vi "Log Tester.vi"() -> ()   [LabVIEW 2015]
uses:
  Controls/QMH Fundamentals - Message Cluster.ctl
  Controls/Config_Stop Notifier Enum.ctl
  Controls/Control_Message Handling Cluster.ctl
  Controls/Control_M4X Connection.ctl
  Controls/Control_PXI-7854R FPGA Reference.ctl
  Controls/Control_Config Cluster.ctl
  Controls/Control_Config Unitherm Port.ctl
  Controls/Control_Config Simulate Values.ctl
  Controls/Control_Log Queue.ctl
  Controls/Control_Log Cluster.ctl
  Controls/Control_Log Time.ctl
  Controls/Control_Log Waveform Cluster.ctl
  Controls/Control_Log Analysis Cluster.ctl
  Controls/Control_Log Flag.ctl
  <vilib>/Waveform/WDTFileIO.llb/ Write Waveform to File.vi
  <vilib>/Waveform/WDTFileIO.llb/Export Waveforms To Spreadsheet File (1D).vi
panel:
  out "Saving Data":bool
  out "Time":timestamp
  in  "Simulate":bool
  out "Logging?":bool
  out "error out":errorcluster
  out "Measurements out":T1
  out "Waveform out":waveform(dbl)
  in  "error in (no error)":errorcluster
  in  "Log?":bool
  in  "Measurements in":T1
  in  "Waveform in":waveform(dbl)
  in  "stop":bool
  # "Real Values"
  # "Simulate"
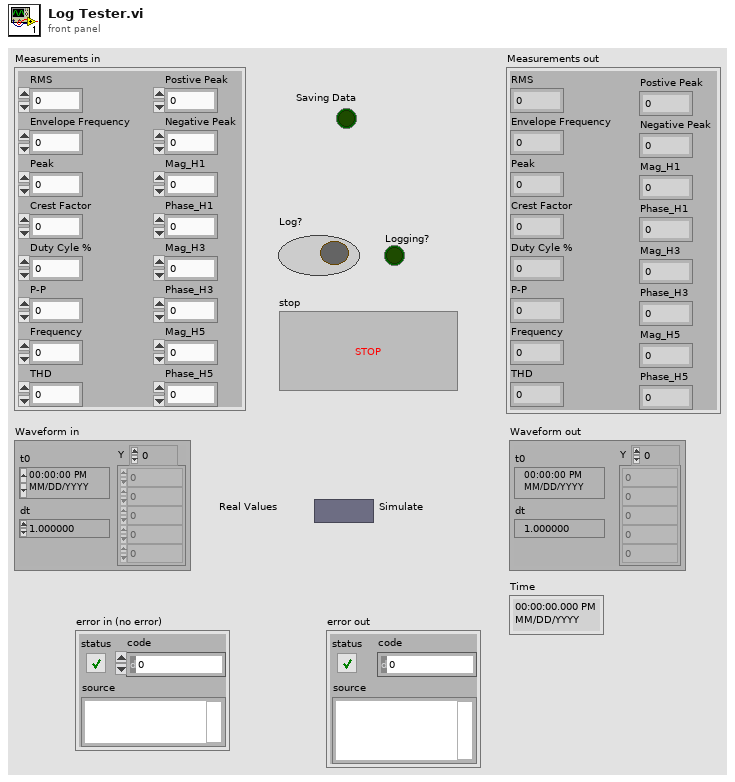
[diagram p1: front panel]
types:
  T1 = cluster{"RMS":dbl, "Envelope Frequency":dbl, "Peak":dbl, "Crest Factor":dbl, "Duty Cyle %":dbl, "P-P":dbl, "Frequency":dbl, "THD":dbl, "Postive Peak":dbl, "Negative Peak":dbl, "Mag_H1":dbl, "Phase_H1":dbl, "Mag_H3":dbl, "Phase_H3":dbl, "Mag_H5":dbl, "Phase_H5":dbl}
  T2 = enum16{"open", "open or create", "create or replace", "create", "open (read-only)"}
  T3 = cluster{"Time":timestamp, "Waveform":waveform(dbl), "Measurements":cluster{"RMS":dbl, "Envelope Frequency":dbl, "Peak":dbl, "Crest Factor":dbl, "Duty Cyle %":dbl, "P-P":dbl, "Frequency":dbl, "THD":dbl, "Postive Peak":dbl, "Negative Peak":dbl, "Mag_H1":dbl, "Phase_H1":dbl, "Mag_H3":dbl, "Phase_H3":dbl, "Mag_H5":dbl, "Phase_H5":dbl}}
  T4 = typedef "Config_Stop Notifier Enum.ctl" = enum16{"Initialize", "Read Notifier", "Notify", "Close"}
  T5 = cluster{"Log":bool, "Card Handle in":u32, "Simulate?":bool, "Measurements":cluster{"RMS":dbl, "Envelope Frequency":dbl, "Peak":dbl, "Crest Factor":dbl, "Duty Cyle %":dbl, "P-P":dbl, "Frequency":dbl, "THD":dbl, "Postive Peak":dbl, "Negative Peak":dbl, "Mag_H1":dbl, "Phase_H1":dbl, "Mag_H3":dbl, "Phase_H3":dbl, "Mag_H5":dbl, "Phase_H5":dbl}, "Waveform":waveform(dbl)}
  T6 = typedef "QMH Fundamentals - Message Cluster.ctl" = cluster{"Message":string, "Message Data":variant}
  T7 = typedef "Control_Message Handling Cluster.ctl" = cluster{"Fornax Connected?":refnum<vi>, "Unitherm Connected?":refnum<vi>, "M4X Connected?":refnum<vi>, "Unitherm Connect/Disconnect":refnum<vi>, "Fornax Connection":refnum<k5>, "UNITHERM Connection":refnum<visa-resource-name>, "M4X Connection":T8, "PXI-7854R FPGA Reference":T9, "PXI-7854R Connected?":refnum<vi>, "Fornax Connect/Disconnect":refnum<vi>, "7854 Connect/Disconnect":refnum<vi>, "M4X Connect/Disconnect":refnum<vi>, "Config Cluster":T10, "Log Queue":T13, "Log Analysis Cluster":T14, "Log Waveform Cluster":T15, "Log Time":T16, "Log Flag":T17}
  T8 = typedef "Control_M4X Connection.ctl" = u32
  T9 = typedef "Control_PXI-7854R FPGA Reference.ctl" = refnum<k20>
  T10 = typedef "Control_Config Cluster.ctl" = cluster{"Unitherm Port":T11, "Simulate Values":T12}
  T11 = typedef "Control_Config Unitherm Port.ctl" = string
  T12 = typedef "Control_Config Simulate Values.ctl" = bool
  T13 = typedef "Control_Log Queue.ctl" = refnum<queue>
  T14 = typedef "Control_Log Analysis Cluster.ctl" = cluster{"RMS":dbl, "Envelope Frequency":dbl, "Peak":dbl, "Crest Factor":dbl, "Duty Cyle %":dbl, "P-P":dbl, "Frequency":dbl, "THD":dbl, "Postive Peak":dbl, "Negative Peak":dbl, "Mag_H1":dbl, "Phase_H1":dbl, "Mag_H3":dbl, "Phase_H3":dbl, "Mag_H5":dbl, "Phase_H5":dbl}
  T15 = typedef "Control_Log Waveform Cluster.ctl" = waveform(dbl)
  T16 = typedef "Control_Log Time.ctl" = timestamp
  T17 = typedef "Control_Log Flag.ctl" = bool
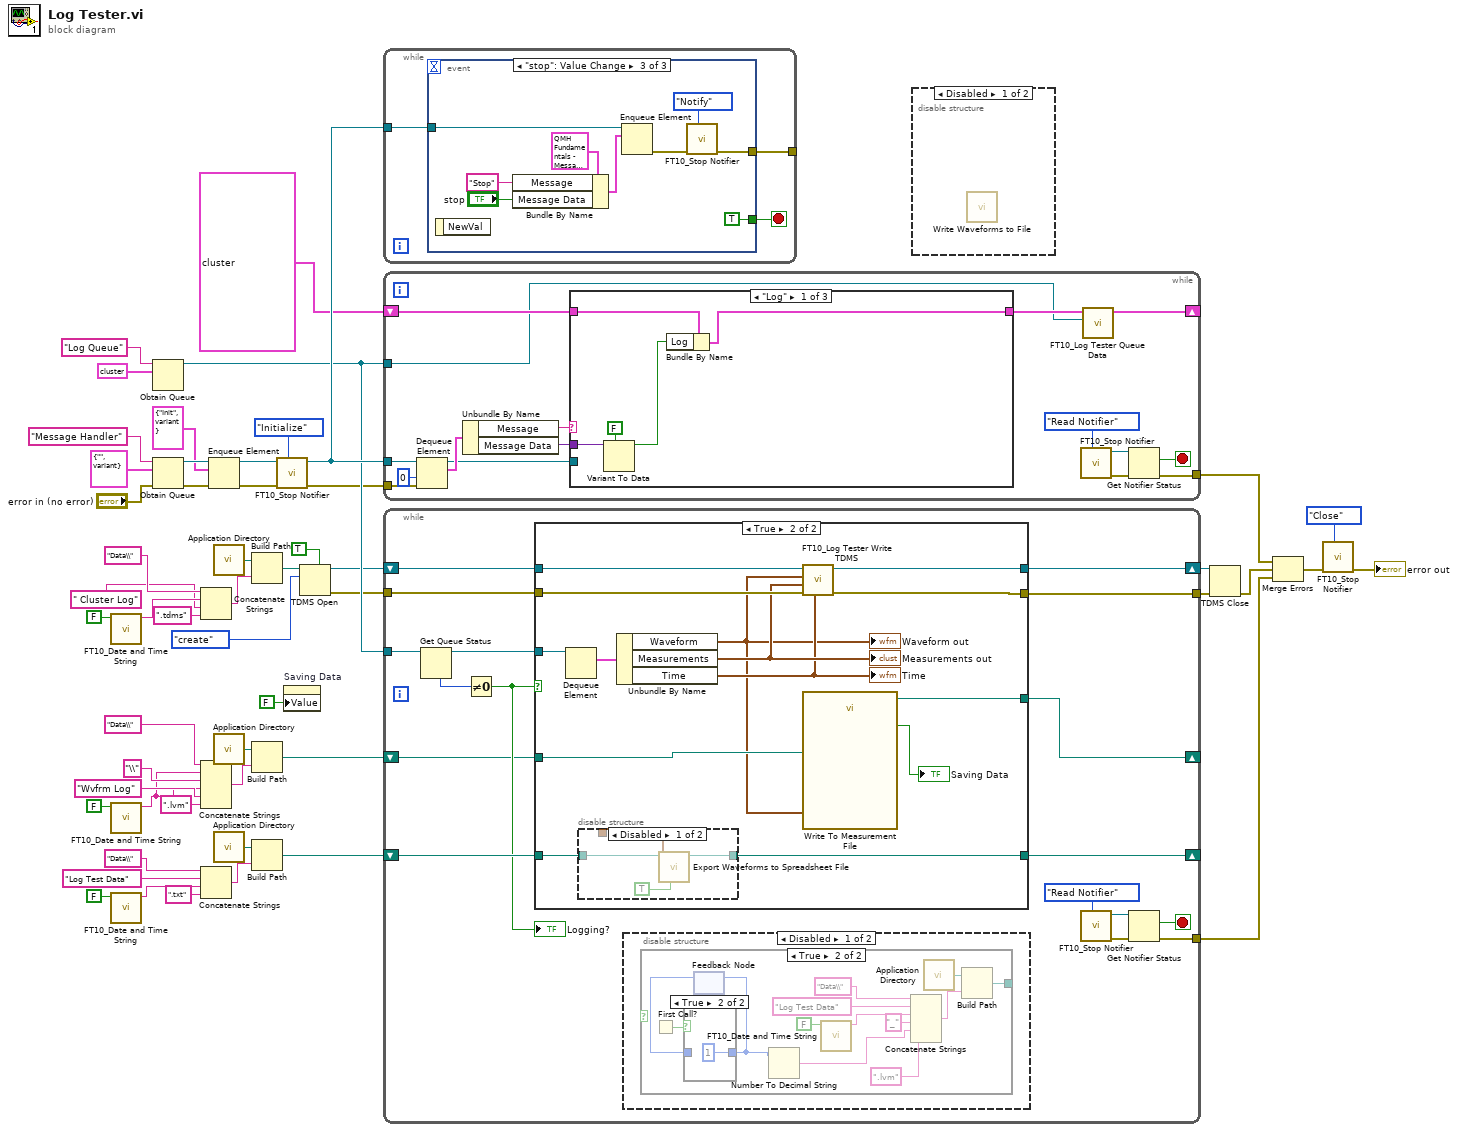
[diagram p0: block diagram]
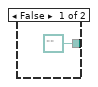
[diagram p3: hidden frame]
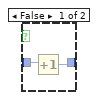
[diagram p4: hidden frame]
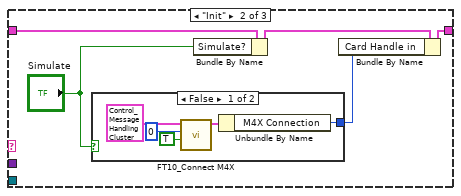
[diagram p8: hidden frame]
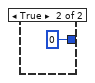
[diagram p9: hidden frame]
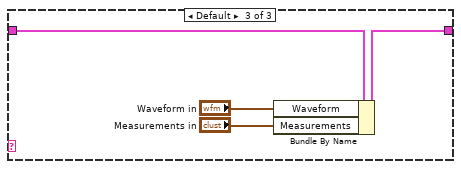
[diagram p10: hidden frame]
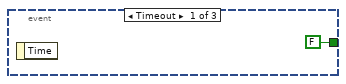
[diagram p11: hidden frame]
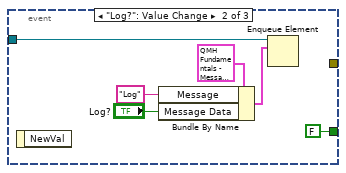
[diagram p12: hidden frame]
diagram:
  n1 = call "FT10_Date and Time String.vi"("to UTC"=FALSE) -> ("Date & Time string"=w4:string)  [unwired: 10 in]
  n2 = call "FT10_Date and Time String.vi"("to UTC"=FALSE) -> ("Date & Time string"=w1:string)  [unwired: 10 in]
  n3 = call "FT10_Date and Time String.vi"("to UTC"=FALSE) -> ("Date & Time string"=w13:string)  [unwired: 10 in]
  n4 = Obtain Queue(name (unnamed)="Log Queue", element data type=T3 {"Time"=timestamp(0 s since 1904-01-01), "Waveform"={"t0"=timestamp(0 s since 1904-01-01), "dt"=1.0, "Y"=[]}, "Measurements"={"RMS"=0.0, "Envelope Frequency"=0.0, "Peak"=0.0, "Crest Factor"=0.0, "Duty Cyle %"=0.0, "P-P"=0.0, "Frequency"=0.0, "THD"=0.0, "Postive Peak"=0.0, "Negative Peak"=0.0, "Mag_H1"=0.0, "Phase_H1"=0.0, "Mag_H3"=0.0, "Phase_H3"=0.0, "Mag_H5"=0.0, "Phase_H5"=0.0}}) -> (queue out=w42:refnum<queue>)  [unwired: 3 in, 2 out]
  n5 = Obtain Queue(name (unnamed)="Message Handler", element data type=T6 {"Message"="", "Message Data"=variant} ("Message Cluster"), error in (no error)="error in (no error)") -> (queue out=w51:refnum<queue>, error out=w48:errorcluster)  [unwired: 2 in, 1 out]
  n6 = Concatenate Strings("Data\\" ("string"), w4, " Cluster Log" ("name or relative path"), ".tdms" ("string")) -> (w24:string)
  n7 = Concatenate Strings("Data\\" ("string"), w1, "\\" ("string"), w1, "Wvfrm Log" ("name or relative path"), ".lvm" ("string")) -> (w20:string)
  n8 = Concatenate Strings("Data\\" ("string"), "Log Test Data" ("name or relative path"), w13, ".txt" ("string")) -> (w14:string)
  n9 = Enqueue Element(queue=w51, element=T6 {"Message"="Init", "Message Data"=variant}, error in (no error)=w48) -> (queue out=w46:refnum<queue>, error out=w44:errorcluster)  [unwired: 1 in, 1 out]
  n10 = call <vilib>:"Application Directory.vi"() -> ("Application Directory"=w30:path)
  n11 = call <vilib>:"Application Directory.vi"() -> ("Application Directory"=w21:path)
  n12 = call <vilib>:"Application Directory.vi"() -> ("Application Directory"=w15:path)
  n13 = Build Path(base path=w30, name or relative path=w24) -> (appended path=w33:path)
  n14 = Build Path(base path=w21, name or relative path=w20) -> (appended path=w8:path)
  n15 = Build Path(base path=w15, name or relative path=w14) -> (appended path=w9:path)
  n16 = call "FT10_Stop Notifier.vi"("Selector"=Config_Stop_Notifier_Enum."Initialize", "error in (no error)"=w44) -> ("error out"=w37:errorcluster)  [unwired: 8 in, 1 out]
  n17 = property on="Saving Data" class="Bool (strict)"("Value"=FALSE ("Saving Data")) -> ()  [unwired: 2 in, 2 out]
  n18 = TDMS Open(5:TRUE ("create index file? (T)"), 10:T2."create" ("operation (0:open)"), 11:w33) -> (0:w29:errorcluster, 3:w32:refnum<k34>)  [unwired: 4 in]
  n19 = while {
    tunnel: w46 -> [w54]
    tunnel: [w53] -> _
    stop <- w55 stop-if-true
    n20 = event shown="[2] \"stop\": Value Change" {
      selector: _ -> [_ _ _]
      dyn-events: _ -> [_ _ _]
      timeout: _ -> [_ _ _]
      tunnel: [FALSE FALSE TRUE] -> w55
      tunnel: w54 -> [_ w61 w67]
      tunnel: [_ _ w64] -> w53
      event Timeout {
        n21 = event-data() -> ()  [unwired: 1 in, 1 out]
      }
      event "Log?": Value Change {
        n22 = event-data() -> ()  [unwired: 1 in, 1 out]
        n23 = Bundle By Name(cluster=T6 {"Message"="Fornax Connect/Disconnect", "Message Data"=variant} ("element"), "Message"="Log", "Message Data"="Log?") -> (w59:T6)
        n24 = Enqueue Element(queue=w61, element=w59) -> ()  [unwired: 2 in, 3 out]
      }
      event "stop": Value Change {
        n25 = event-data() -> ()  [unwired: 1 in, 1 out]
        n26 = Bundle By Name(cluster=T6 {"Message"="Fornax Connect/Disconnect", "Message Data"=variant} ("element"), "Message"="Stop", "Message Data"="stop") -> (w69:T6)
        n27 = Enqueue Element(queue=w67, element=w69) -> (error out=w65:errorcluster)  [unwired: 2 in, 2 out]
        n28 = call "FT10_Stop Notifier.vi"("Selector"=Config_Stop_Notifier_Enum."Notify", "error in (no error)"=w65) -> ("error out"=w64:errorcluster)  [unwired: 8 in, 1 out]
      }
    }
  }
  n29 = while {
    tunnel: w46 -> [w86]
    shift-right: [w73] -> _
    shift-left: T5 {"Log"=FALSE, "Card Handle in"=0, "Simulate?"=FALSE, "Measurements"={"RMS"=0.0, "Envelope Frequency"=0.0, "Peak"=0.0, "Crest Factor"=0.0, "Duty Cyle %"=0.0, "P-P"=0.0, "Frequency"=0.0, "THD"=0.0, "Postive Peak"=0.0, "Negative Peak"=0.0, "Mag_H1"=0.0, "Phase_H1"=0.0, "Mag_H3"=0.0, "Phase_H3"=0.0, "Mag_H5"=0.0, "Phase_H5"=0.0}, "Waveform"={"t0"=timestamp(0 s since 1904-01-01), "dt"=1.0, "Y"=[]}} -> [w82]
    tunnel: w37 -> [w81]
    tunnel: w42 -> [w72]
    tunnel: [w76] -> w38
    stop <- w75 stop-if-true
    n30 = Dequeue Element(queue=w86, timeout in ms (-1)=0, error in (no error)=w81) -> (queue out=w83:refnum<queue>, element=w87:T6)  [unwired: 2 out]
    n31 = Unbundle By Name(w87) -> ("Message"=w85:string, "Message Data"=w84:variant)
    n32 = case shown="\"Log\"" w85 {
      tunnel: w84 -> [w92 _ _]
      tunnel: w83 -> [_ _ _]
      tunnel: [w90 w94 w106] -> w74
      tunnel: w82 -> [w89 w97 w107]
      frame "Log" {
        n33 = Variant To Data(type=FALSE, Variant=w92) -> (data=w88:bool)  [unwired: 1 in, 1 out]
        n34 = Bundle By Name(cluster=w89, "Log"=w88) -> (w90:T5)
      }
      frame "Init" {
        n35 = case shown="False" "Simulate" {
          tunnel: [w98 T8 0 ("M4X Connection")] -> w93
          frame False {
            n36 = call "FT10_Connect M4X.vi"("reset device"=TRUE, "Board #"=u32 0, "Message Handling Cluster in"=T7 {"Fornax Connected?"=refnum, "Unitherm Connected?"=refnum, "M4X Connected?"=refnum, "Unitherm Connect/Disconnect"=refnum, "Fornax Connection"=refnum, "UNITHERM Connection"="", "M4X Connection"=0, "PXI-7854R FPGA Reference"=refnum, "PXI-7854R Connected?"=refnum, "Fornax Connect/Disconnect"=refnum, "7854 Connect/Disconnect"=refnum, "M4X Connect/Disconnect"=refnum, "Config Cluster"={"Unitherm Port"="COM4", "Simulate Values"=TRUE}, "Log Queue"=refnum, "Log Analysis Cluster"={"RMS"=0.0, "Envelope Frequency"=0.0, "Peak"=0.0, "Crest Factor"=0.0, "Duty Cyle %"=0.0, "P-P"=0.0, "Frequency"=0.0, "THD"=0.0, "Postive Peak"=0.0, "Negative Peak"=0.0, "Mag_H1"=0.0, "Phase_H1"=0.0, "Mag_H3"=0.0, "Phase_H3"=0.0, "Mag_H5"=0.0, "Phase_H5"=0.0}, "Log Waveform Cluster"={"t0"=timestamp(0 s since 1904-01-01), "dt"=1.0, "Y"=[]}, "Log Time"=timestamp(0 s since 1904-01-01), "Log Flag"=FALSE}) -> ("Message Handling Cluster out"=w102:T7)  [unwired: 5 in, 3 out]
            n37 = Unbundle By Name(w102) -> ("M4X Connection"=w98:T8)
          }
          frame True {
          }
        }
        n38 = Bundle By Name(cluster=w97, "Simulate?"="Simulate") -> (w96:T5)
        n39 = Bundle By Name(cluster=w96, "Card Handle in"=w93) -> (w94:T5)
      }
      frame Default {
        n40 = Bundle By Name(cluster=w107, "Waveform"="Waveform in", "Measurements"="Measurements in") -> (w106:T5)
      }
    }
    n41 = call "FT10_Stop Notifier.vi"("Selector"=Config_Stop_Notifier_Enum."Read Notifier") -> ("error out"=w77:errorcluster, "Notifier out"=w78:refnum<notifier>)  [unwired: 9 in]
    n42 = call "FT10_Log Tester Queue Data.vi"("Queue in"=w72, "Cluster in"=w74) -> ("Cluster out"=w73:T5)  [unwired: 9 in]
    n43 = Get Notifier Status(notifier=w78, error in (no error)=w77) -> (current notification=w75:bool, error out=w76:errorcluster)  [unwired: 3 out]
  }
  n44 = while {
    tunnel: w42 -> [w124]
    tunnel: [w119] -> w25
    shift-right: [w115] -> w28
    shift-left: w32 -> [w116]
    tunnel: w29 -> [w114]
    tunnel: [w113] -> w27
    shift-right: [w110] -> _
    shift-left: w8 -> [w108]
    shift-right: [w111] -> _
    shift-left: w9 -> [w112]
    stop <- w120 stop-if-true
    n45 = Get Queue Status(queue=w124) -> (queue out=w118:refnum<queue>, # elements in queue=w117:i32)  [unwired: 2 in, 6 out]
    n46 = Not Equal To 0?(x=w117) -> (x != 0?=w109:bool)
    "Logging?" <- w109
    n47 = case shown="True" w109 {
      tunnel: w118 -> [_ w159]
      tunnel: w116 -> [w145 w157]
      tunnel: [w145 w156] -> w115
      tunnel: w114 -> [w144 w155]
      tunnel: [w144 w154] -> w113
      tunnel: w108 -> [w143 w151]
      tunnel: [w143 w146] -> w110
      tunnel: w112 -> [w142 w149]
      tunnel: [w142 w148] -> w111
      frame False {
      }
      frame True {
        n48 = Dequeue Element(queue=w159) -> (element=w158:T3)  [unwired: 2 in, 3 out]
        n49 = disable-structure shown="Disabled" {
          disable-tunnel: w149 -> [w163 w164]
          disable-tunnel: [w162 w164] -> w148
          disable-tunnel: _ -> [w160 _]
          frame Disabled {
            n50 = call-poly <vilib>:"Export Waveforms to Spreadsheet File.vi"("append to file? (new file:F)"=TRUE, "waveforms"=w160, "file path (dialog if empty)"=w163) -> ("new file path (Not A Path if cancelled)"=w162:path)  [unwired: 7 in, 1 out]
          }
          frame Enabled {
          }
        }
        n51 = Unbundle By Name(w158) -> ("Waveform"=w147:waveform(dbl), "Measurements"=w153:T1, "Time"=w152:timestamp)
        "Waveform out" <- w147
        "Measurements out" <- w153
        "Time" <- w152
        n52 = call "FT10_Log Tester Write TDMS.vi"("Time in"=w152, "error in (no error)"=w155, "Measurements in"=w153, "Waveform in"=w147, "Refnum in"=w157) -> ("error out"=w154:errorcluster, "Refnum out"=w156:refnum<k34>)  [unwired: 5 in]
        n53 = call "Write To Measurement File"("Signals"=w147, "Filename"=w151) -> ("Filename Out"=w146:path, "Saving Data"=→"Saving Data":bool)  [unwired: 15 in, 1 out]
      }
    }
    n54 = disable-structure shown="Disabled" {
      frame Disabled {
        n55 = case shown="True" {
          selector: _ -> [_ _]
          tunnel: [path "" ("appended path") w126] -> _
          frame False {
          }
          frame True {
            n56 = First Call?() -> (First Call?: T/F=w130:bool)
            n57 = feedback #1() -> (w129:i32)  [unwired: 1 in]
            n58 = case shown="True" w130 {
              tunnel: [w139 1] -> w128
              tunnel: w129 -> [w140 _]
              frame False {
                n59 = Increment(x=w140) -> (x+1=w139:i32)
              }
              frame True {
              }
            }
            n60 = feedback-in #1(w128) -> ()
            n61 = Number To Decimal String(number=w128) -> (decimal integer string=w127:string)  [unwired: 1 in]
            n62 = call "FT10_Date and Time String.vi"("to UTC"=FALSE) -> ("Date & Time string"=w135:string)  [unwired: 10 in]
            n63 = Concatenate Strings("Data\\" ("string"), "Log Test Data" ("name or relative path"), w135, "_" ("string"), w127, ".lvm" ("string")) -> (w136:string)
            n64 = call <vilib>:"Application Directory.vi"() -> ("Application Directory"=w137:path)
            n65 = Build Path(base path=w137, name or relative path=w136) -> (appended path=w126:path)
          }
        }
      }
      frame Enabled {
      }
    }
    n66 = call "FT10_Stop Notifier.vi"("Selector"=Config_Stop_Notifier_Enum."Read Notifier") -> ("error out"=w121:errorcluster, "Notifier out"=w122:refnum<notifier>)  [unwired: 9 in]
    n67 = Get Notifier Status(notifier=w122, error in (no error)=w121) -> (current notification=w120:bool, error out=w119:errorcluster)  [unwired: 3 out]
  }
  n68 = disable-structure shown="Disabled" {
    frame Disabled {
      n69 = call-poly <vilib>:"Write Waveforms to File.vi"() -> ()  [unwired: 10 in, 2 out]
    }
    frame Enabled {
    }
  }
  n70 = TDMS Close(8:w27, 11:w28) -> (0:w26:errorcluster)  [unwired: 1 out]
  n71 = Merge Errors(w38, w26, w25) -> (w39:errorcluster)
  n72 = call "FT10_Stop Notifier.vi"("Selector"=Config_Stop_Notifier_Enum."Close", "error in (no error)"=w39) -> ("error out"=→"error out":errorcluster)  [unwired: 8 in, 1 out]
